vi "timeout_UDP (SubVI).vi"(11 "length":i32) -> (3 "timeout UDP":i32)   [LabVIEW 2017]
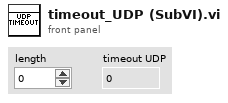
[diagram p1: front panel]
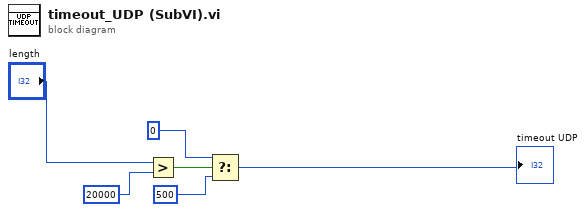
[diagram p0: block diagram]
diagram:
  n1 = Greater?(x="length", y=20000) -> (0:w2:bool)
  n2 = Select(t=0, s=w2, f=500 ("t")) -> (s? t:f=→"timeout UDP":i32)
